vi "2016RefLoopPulseGen_Cleaned.vi"() -> ()   [LabVIEW 2017]
uses:
  <vilib>/Utility/error.llb/DialogType.ctl
  <vilib>/DAQmx/write.llb/DAQmx Write (Digital 1D Bool NChan 1Samp 1Line).vi
  <vilib>/DAQmx/read.llb/DAQmx Read (Analog 1D DBL NChan 1Samp).vi
  <vilib>/DAQmx/write.llb/DAQmx Write (Digital 1D Bool 1Chan 1Samp).vi
  <vilib>/DAQmx/miscellaneous.llb/DAQmx Fill In Error Info.vi
  <vilib>/express/express shared/transition.llb/Dynamic To Waveform Array.vi
  <vilib>/express/express arith-compare/Formula/Block/exnFormulaBlock how many pts in the wave.vi
  <vilib>/express/express shared/ex_Modify Signal Name.vi
  <vilib>/express/express shared/transition.llb/Waveform Array To Dynamic.vi
  <vilib>/DAQmx/create/channels.llb/DAQmx Create Channel (CO-Pulse Generation-Frequency).vi
  <vilib>/DAQmx/configure/timing.llb/DAQmx Timing (Implicit).vi
  <vilib>/DAQmx/configure/timing.llb/DAQmx Timing (Sample Clock).vi
  <vilib>/express/express signal manip/GetorSetDDTAttributes/Set DDT Attributes/SetT0.vi
  <vilib>/express/express arith-compare/Formula/XNode/ExpressFormulaBlockNode.xnode
  <vilib>/express/express signal manip/GetorSetDDTAttributes/Set DDT Attributes/Set DDT Properties.xnode
  <vilib>/addons/control/pid/NI_PID_autopid.lvlib
panel:
  in  "stop 4":bool
  in  "?":bool
  out "error out 2":errorcluster
  out "error out":errorcluster
  in  "output duty cycle range 1":cluster{"output high":dbl, "output low":dbl}={"output high"=100.0, "output low"=0.0}
  out "Waveform Chart":dbl(graph)=1.0280585289001465
  out "Elapsed Time (s)":dbl=1192.0481810569763
  in  "?":T1(tab)
  in  "Lower Test Section offset":dbl
  in  "Vapor Inlet T offset":dbl
  in  "Liquid Tank P offset":dbl=8500.0
  out "Test Section P (Pa)":dbl=116198.57530062649
  in  "P atm":dbl=101325.0
  in  "Liquid Inlet Offset":dbl=1100.0
  in  "Upper Test Sec":dbl
  in  "Dev Section P offset":dbl=-15000.0
  in  "Liquid Inlet T offset":dbl
  in  "Separator T offset":dbl
  in  "Liquid Tank T offset":dbl
  in  "Vapor Tank T offset":dbl
  in  "Separator P Offset":dbl=2500.0
  out "dP [Pa]  W1 to W7":dbl=-0.008208439355650089
  out "dP [Pa] W1 to W4":dbl=0.008075495341450085
  out "Liquid Tank Heater Temp. [C]":dbl=-0.00013997779130803294 format="%#_4g"
  out "Vapor Tank Heater Temp. [C]":dbl=-0.00010921620483495026 format="%#_4g"
  in  "Vapor Tank Heater [V]":dbl(slide) scale=0.0..10.0
  in  "Liquid Tank Heater [V]":dbl(slide) scale=0.0..10.0
  out "Quality\n[-]":dbl=0.5124735258578829 format="%#_3f"
  out "Mixture Enthalpy":dbl=315341.8738601937
  out "Upper TS Sat. Temp. [C]":dbl=-30.741985921320232 format="%#_4g"
  out "Upper Test Section 2\n(not connected)":dbl=19080.10707676887
  out "?":dbl=nan format="%#_4g"
  out "?":dbl=nan format="%#_4g"
  out "Vapor Inlet Sat. Temp. [C]":dbl=18.983650599672455 format="%#_4g"
  out "Liquid Inlet Sat. Temp. [C]":dbl=18.967113726868046 format="%#_4g"
  out "Separator Sat. Temp. [C]":dbl=18.962084458713754 format="%#_4g"
  out "Liquid Tank Sat. Temp. [C]":dbl=17.336038014955804 format="%#_4g"
  out "Vapor Tank Sat. Temp. [C]":dbl=nan format="%#_4g"
  out "Lower Test Section 2\n(not connected)":dbl=-5.945274707393333 format="%#_6f"
  out "Streamwise":dbl=-4309.180034596612 format="%#_2e"
  out "Dev Section":dbl=117529.39865406745 format="%#_5f"
  out "Separator 2":dbl=117436.76445279745 format="%#_5f"
  out "Vapor Tank 2\n(need replaced)":dbl=-34009.73110511369 format="%#_6f"
  out "Liquid Inlet 2":dbl=117458.36040777806 format="%#_5f"
  out "Liquid Tank 2":dbl=119158.55398835387 format="%#_5f"
  out "Upper TS Sat. Pres.":dbl=117745.79282373996
  out "Upper Test Section":dbl=19.02953821278611 format="%#_4g"
  out "Lower Test Section":dbl=18.841711969674257 format="%#_4g"
  out "Vapor Inlet":dbl=19.940090617924646 format="%#_4g"
  out "Liquid Inlet":dbl=19.29273815741822 format="%#_4g"
  out "Separator":dbl=19.351746784304748 format="%#_4g"
  out "Liquid Tank":dbl=19.064732737324512 format="%#_4g"
  out "Vapor Tank":dbl=19.311251471245498 format="%#_4g"
  out "Liquid Inlet Sat. Pres.":dbl=118921.18754866866 format="%#_4f"
  out "Liquid Tank Sat. Pres.":dbl=117902.28866165497 format="%#_4f"
  out "Vapor Inlet Sat. Pres.":dbl=119186.31350697557 format="%#_4f"
  out "Lower Test Section Sat. Pres.":dbl=116914.11104502712 format="%#_4f"
  out "Separator Sat. Pres.":dbl=121862.28710047182 format="%#_4f"
  out "Vapor Tank Sat. Pres.":dbl=119004.3043776936 format="%#_4f"
  out "Evaporator Bottom":dbl=0.07812510710210246 format="%#_4g"
  out "Evaporator Top":dbl=-55440.10937765434 format="%#_4g"
  out "Condenser Bottom":dbl=-0.00013633631982423782 format="%#_4g"
  out "Condenser Top":dbl=-0.0001304783004807413 format="%#_4g"
  in  "Save File":bool
  out "StaticPressDiff(Pa)":dbl=-222.00009683752145
  out "DC":dbl
  out "Vapor Mass Flow Current":dbl=2.098083621149279e-08
  out "Pressure Drop":dbl=2.6226045264365988e-08
  in  "Boolean 2":bool
  out "Waveform Chart 2":dynamicdata(graph)
  in  "Pitot Offset [Pa]":dbl
  in  "PG-TS Offset\n[Pa]":dbl
  in  "Send Pulse 2":bool
  out "Psat liq":dbl=119.96937909943745
  in  "Save Loop Data":bool
  in  "Boolean":bool
  in  "Sampling frequency (Hz)":dbl=1000.0
  in  "Length of recording (s)":dbl=2.0
  in  "PG Abs Offset":dbl=11500.0
  out "Psat vap":dbl=121.24568157832624
  out "Pitot Amps":dbl=2.6415199999999147e-07
  out "dP Pitot Probe":dynamicdata(graph)=[{"t0"=timestamp(3554308544.5452676 s since 1904-01-01), "dt"=0.001, "Y"=array[2000 elements], "attributes"=variant("NI_ChannelName"=variant(string "Pitot dP (Formula Result)"), "NI_OriginalChannelName"=variant(string "Pitot dP"), "NI_UnitDescription"=variant(string "Amps"))}]
  out "Tank Pressure":dynamicdata(graph)=[{"t0"=timestamp(3554308544.5452676 s since 1904-01-01), "dt"=0.001, "Y"=array[2000 elements], "attributes"=variant("NI_ChannelName"=variant(string "Abs P (Formula Result)"), "NI_OriginalChannelName"=variant(string "Abs P"), "NI_UnitDescription"=variant(string "Volts"))}]
  out "dP to test section":dynamicdata(graph)=[{"t0"=timestamp(3554308544.5452814 s since 1904-01-01), "dt"=0.001, "Y"=array[2000 elements], "attributes"=variant("NI_ChannelName"=variant(string "PG to TS dP (Formula Result)"), "NI_OriginalChannelName"=variant(string "PG to TS dP"), "NI_UnitDescription"=variant(string "Volts"))}]
  out "Pitot dP":dbl=-4308.9404273994505
  out "Liquid Temp":dbl=19.52526901660894
  out "Vapor Temp":dbl=19.805676371442082
  in  "CCW":bool
  in  "?":bool
  out "Loop iterations":i32
  in  "Send Pulse":bool
  in  "Steps":i32=10000 min=0 max=40000 step=500
  in  "Idle State":i32(ring)=10214 items=["High"=10192, "Low"=10214]
  in  "Counter(s)":tag="cDAQ1Mod8/ctr0" caption="Counter"
  in  "Duty Cycle":dbl=0.5 min=0.1 max=1.0 step=0.1
  in  "Frequency (Hz)":dbl=1000.0 min=0.0 max=10000.0 step=500.0
  out "Mass Flow Rate":dbl=nan
  in  "Heaters":bool
  out "PG Abs":dbl=119484.80284900061
  out "PG to TS dP":dbl=4351.8068090218785
  in  "Save dP data":bool
  in  "Vapor Flow Set Point [g/s]":dbl format="%.2f"
  in  "stop":bool
  in  "reinitialize? (F) 2":bool=TRUE
  out "Liquid Mass Flow Rate":cluster{"[0]":dbl, "[1]":dbl}(graph)={"[0]"=0.0, "[1]"=-94.2977673785965}
  out "Voltage Out 2":dbl
  out "Liquid Line Density [g/cm3]":dbl=-0.5000013113022632
  out "Liquid Flow Rate [g/s]":dbl=-94.2977673785965
  in  "LiquidOnOff":bool
  in  "LiquidManPID":bool
  in  "PID gains 2":T2={"proportional gain (Kc)"=1e-15, "integral time (Ti, min)"=1e-12, "derivative time (Td, min)"=1e-12} {"derivative time (Td, min)" format="%.4e"; "integral time (Ti, min)" format="%.4e"; "proportional gain (Kc)" format="%.4e"}
  in  "output range 2":cluster{"output high":dbl, "output low":dbl}={"output high"=4.5, "output low"=2.0} {"output low" format="%.2f"; "output high" format="%.2f"}
  in  "Valve Voltage [V] 2":dbl=2.6 format="%.2f"
  in  "Liquid Flow Set Point\n[g/s]":dbl format="%.2f"
  in  "output range":cluster{"output high":dbl, "output low":dbl}={"output high"=3.0, "output low"=2.0} {"output low" format="%.2f"; "output high" format="%.2f"}
  in  "PID gains":T2={"proportional gain (Kc)"=1e-14, "integral time (Ti, min)"=1e-12, "derivative time (Td, min)"=1e-12} {"derivative time (Td, min)" format="%.4e"; "integral time (Ti, min)" format="%.4e"; "proportional gain (Kc)" format="%.4e"}
  in  "VaporManPID":bool
  in  "VaporOnOff":bool
  in  "Valve Voltage [V]":dbl=2.33 format="%.2f"
  out "Vapor Line Density [g/cm3]":dbl=-0.5000029504300922
  out "Vapor Flow Rate [g/s]":dbl=-94.29782933653023
  out "Voltage Out":dbl
  out "Vapor Mass Flow Rate":cluster{"[0]":dbl, "[1]":dbl}(graph)
  in  "reinitialize? (F)":bool=TRUE
  in  "PID on 2":bool
  in  "T1 Setpoint [C]":dbl format="%.2f"
  in  "reinitialize? (F) 3":bool=TRUE
  in  "PID gains 3":T2={"proportional gain (Kc)"=1e-14, "integral time (Ti, min)"=1e-12, "derivative time (Td, min)"=1e-12} {"derivative time (Td, min)" format="%.4e"; "integral time (Ti, min)" format="%.4e"; "proportional gain (Kc)" format="%.4e"}
  out "T1":cluster{"[0]":dbl, "[1]":dbl}(graph)
  out "T1 Measured [C]":dbl
  out "DutyCycleCalc1":dbl format="%.6f"
  in  "T2 Setpoint [C]":dbl format="%.2f"
  in  "reinitialize? (F) 4":bool=TRUE
  in  "PID gains 4":T2={"proportional gain (Kc)"=1e-14, "integral time (Ti, min)"=1e-12, "derivative time (Td, min)"=1e-12} {"derivative time (Td, min)" format="%.4e"; "integral time (Ti, min)" format="%.4e"; "proportional gain (Kc)" format="%.4e"}
  out "T2":cluster{"[0]":dbl, "[1]":dbl}(graph)
  out "T2 Measured [C]":dbl
  out "DutyCycleCalc2":dbl format="%.6f"
  in  "stop 2":bool
  in  "PID on":bool
  in  "PID on 3":bool
  in  "T3 Setpoint [C]":dbl format="%.2f"
  in  "reinitialize? (F) 5":bool=TRUE
  in  "PID gains 5":T2={"proportional gain (Kc)"=1e-14, "integral time (Ti, min)"=1e-12, "derivative time (Td, min)"=1e-12} {"derivative time (Td, min)" format="%.4e"; "integral time (Ti, min)" format="%.4e"; "proportional gain (Kc)" format="%.4e"}
  out "T3":cluster{"[0]":dbl, "[1]":dbl}(graph)
  out "T3 Measured [C]":dbl
  out "DutyCycleCalc3":dbl format="%.6f"
  in  "PID on 4":bool
  in  "T4 Setpoint [C]":dbl format="%.2f"
  in  "reinitialize? (F) 6":bool=TRUE
  in  "PID gains 6":T2={"proportional gain (Kc)"=1e-14, "integral time (Ti, min)"=1e-12, "derivative time (Td, min)"=1e-12} {"derivative time (Td, min)" format="%.4e"; "integral time (Ti, min)" format="%.4e"; "proportional gain (Kc)" format="%.4e"}
  out "T4":cluster{"[0]":dbl, "[1]":dbl}(graph)
  out "T4 Measured [C]":dbl
  out "DutyCycleCalc4":dbl format="%.6f"
  in  "PID on 5":bool
  in  "T5 Setpoint [C]":dbl format="%.2f"
  in  "reinitialize? (F) 7":bool=TRUE
  in  "PID gains 7":T2={"proportional gain (Kc)"=1e-14, "integral time (Ti, min)"=1e-12, "derivative time (Td, min)"=1e-12} {"derivative time (Td, min)" format="%.4e"; "integral time (Ti, min)" format="%.4e"; "proportional gain (Kc)" format="%.4e"}
  out "T5":cluster{"[0]":dbl, "[1]":dbl}(graph)
  out "T5 Measured [C]":dbl
  out "DutyCycleCalc5":dbl format="%.6f"
  in  "PID on 6":bool
  in  "T6 Setpoint [C]":dbl format="%.2f"
  in  "reinitialize? (F) 8":bool=TRUE
  in  "PID gains 8":T2={"proportional gain (Kc)"=1e-14, "integral time (Ti, min)"=1e-12, "derivative time (Td, min)"=1e-12} {"derivative time (Td, min)" format="%.4e"; "integral time (Ti, min)" format="%.4e"; "proportional gain (Kc)" format="%.4e"}
  out "T6":cluster{"[0]":dbl, "[1]":dbl}(graph)
  out "T6 Measured [C]":dbl
  out "DutyCycleCalc6":dbl format="%.6f"
  in  "PID on 7":bool
  in  "T7 Setpoint [C]":dbl format="%.2f"
  in  "reinitialize? (F) 9":bool=TRUE
  in  "PID gains 9":T2={"proportional gain (Kc)"=1e-14, "integral time (Ti, min)"=1e-12, "derivative time (Td, min)"=1e-12} {"derivative time (Td, min)" format="%.4e"; "integral time (Ti, min)" format="%.4e"; "proportional gain (Kc)" format="%.4e"}
  out "T7":cluster{"[0]":dbl, "[1]":dbl}(graph)
  out "T7 Measured [C]":dbl
  out "DutyCycleCalc7":dbl format="%.6f"
  out "WinOn 2":bool
  out "WinOn 1":bool
  in  "PID on 8":bool
  in  "T8 Setpoint [C]":dbl format="%.2f"
  in  "reinitialize? (F) 10":bool=TRUE
  in  "PID gains 10":T2={"proportional gain (Kc)"=1e-14, "integral time (Ti, min)"=1e-12, "derivative time (Td, min)"=1e-12} {"derivative time (Td, min)" format="%.4e"; "integral time (Ti, min)" format="%.4e"; "proportional gain (Kc)" format="%.4e"}
  out "T8":cluster{"[0]":dbl, "[1]":dbl}(graph)
  out "T8 Measured [C]":dbl
  out "DutyCycleCalc8":dbl format="%.6f"
  in  "PID on 9":bool
  in  "T9 Setpoint [C]":dbl format="%.2f"
  in  "reinitialize? (F) 11":bool=TRUE
  in  "PID gains 11":T2={"proportional gain (Kc)"=1e-14, "integral time (Ti, min)"=1e-12, "derivative time (Td, min)"=1e-12} {"derivative time (Td, min)" format="%.4e"; "integral time (Ti, min)" format="%.4e"; "proportional gain (Kc)" format="%.4e"}
  out "T9":cluster{"[0]":dbl, "[1]":dbl}(graph)
  out "T9 Measured [C]":dbl
  out "DutyCycleCalc9":dbl format="%.6f"
  in  "PID on 10":bool
  in  "T10 Setpoint [C]":dbl format="%.2f"
  in  "reinitialize? (F) 12":bool=TRUE
  in  "PID gains 12":T2={"proportional gain (Kc)"=1e-14, "integral time (Ti, min)"=1e-12, "derivative time (Td, min)"=1e-12} {"derivative time (Td, min)" format="%.4e"; "integral time (Ti, min)" format="%.4e"; "proportional gain (Kc)" format="%.4e"}
  out "T10":cluster{"[0]":dbl, "[1]":dbl}(graph)
  out "T10 Measured [C]":dbl
  out "DutyCycleCalc10":dbl format="%.6f"
  in  "PID on 11":bool
  in  "T11 Setpoint [C]":dbl format="%.2f"
  in  "reinitialize? (F) 13":bool=TRUE
  in  "PID gains 13":T2={"proportional gain (Kc)"=1e-14, "integral time (Ti, min)"=1e-12, "derivative time (Td, min)"=1e-12} {"derivative time (Td, min)" format="%.4e"; "integral time (Ti, min)" format="%.4e"; "proportional gain (Kc)" format="%.4e"}
  out "T11":cluster{"[0]":dbl, "[1]":dbl}(graph)
  out "T11 Measured [C]":dbl
  out "DutyCycleCalc11":dbl format="%.6f"
  in  "PID on 12":bool
  in  "T12 Setpoint [C]":dbl format="%.2f"
  in  "reinitialize? (F) 14":bool=TRUE
  in  "PID gains 14":T2={"proportional gain (Kc)"=1e-14, "integral time (Ti, min)"=1e-12, "derivative time (Td, min)"=1e-12} {"derivative time (Td, min)" format="%.4e"; "integral time (Ti, min)" format="%.4e"; "proportional gain (Kc)" format="%.4e"}
  out "T12":cluster{"[0]":dbl, "[1]":dbl}(graph)
  out "T12 Measured [C]":dbl
  out "DutyCycleCalc12":dbl format="%.6f"
  in  "PID on 13":bool
  in  "T13 Setpoint [C]":dbl format="%.2f"
  in  "reinitialize? (F) 15":bool=TRUE
  in  "PID gains 15":T2={"proportional gain (Kc)"=1e-14, "integral time (Ti, min)"=1e-12, "derivative time (Td, min)"=1e-12} {"derivative time (Td, min)" format="%.4e"; "integral time (Ti, min)" format="%.4e"; "proportional gain (Kc)" format="%.4e"}
  out "T13":cluster{"[0]":dbl, "[1]":dbl}(graph)
  out "T13 Measured [C]":dbl
  out "DutyCycleCalc13":dbl format="%.6f"
  in  "PID on 14":bool
  in  "T14 Setpoint [C]":dbl format="%.2f"
  in  "reinitialize? (F) 16":bool=TRUE
  in  "PID gains 16":T2={"proportional gain (Kc)"=1e-14, "integral time (Ti, min)"=1e-12, "derivative time (Td, min)"=1e-12} {"derivative time (Td, min)" format="%.4e"; "integral time (Ti, min)" format="%.4e"; "proportional gain (Kc)" format="%.4e"}
  out "T14":cluster{"[0]":dbl, "[1]":dbl}(graph)
  out "T14 Measured [C]":dbl
  out "DutyCycleCalc14":dbl format="%.6f"
  # "Same button as Save data loop button on Pulse Generator tab"
  # "Test Section Properties"
  # "Pressure\n[Pa]"
  # "Sat. Temp.\n[C]"
  # "Sat. Pressure\n[Pa]"
  # "Temp.\n[C]"
  # "Temperature [C]"
  # "Condenser"
  # "Evaporator"
  # "Top"
  # "Bottom"
  # "Save File"
  # "Do Not\nSave File"
  # "In order to send a  group of pulses follow the steps below.\n1)Press the button labeled Send Pulse\n2)Press the button a second time in order to prepare for another pulse\n3)Press the stop button to reset the Send Pulse button\n4)Repeat process for next pulse\n\nNote: 1000 steps is a full cycle of the valve, this will send one pulse"
  # "Saving Data:\n\n- Press the Save Loop Data button to record time-averaged (every 2s) data from the loop (data from Test Section Properties tab). Pressing the button again keeps writing in the same file.\n\n-Press the Save dP data to record time resolved data. Each time you press the button, a new file is recorded."
  # "Pulse Generator\nTemperatures"
  # "Vapor Side"
  # "Valve On"
  # "Valve Off"
  # "Manual Flow\nControl"
  # "PID Flow\nControl"
  # "Liquid Side"
  # "Valve On"
  # "Valve Off"
  # "Manual Flow\nControl"
  # "PID Flow\nControl"
  # "Heater On"
  # "Heater On"
  # "Heater On"
  # "Heater On"
  # "Heater Off"
  # "Heater Off"
  # "Heater Off"
  # "Heater Off"
  # "Heater On"
  # "Heater On"
  # "Heater On"
  # "Heater Off"
  # "Heater Off"
  # "Heater Off"
  # "Heater On"
  # "Heater On"
  # "Heater On"
  # "Heater On"
  # "Heater Off"
  # "Heater Off"
  # "Heater Off"
  # "Heater Off"
  # "Heater On"
  # "Heater On"
  # "Heater On"
  # "Heater Off"
  # "Heater Off"
  # "Heater Off"
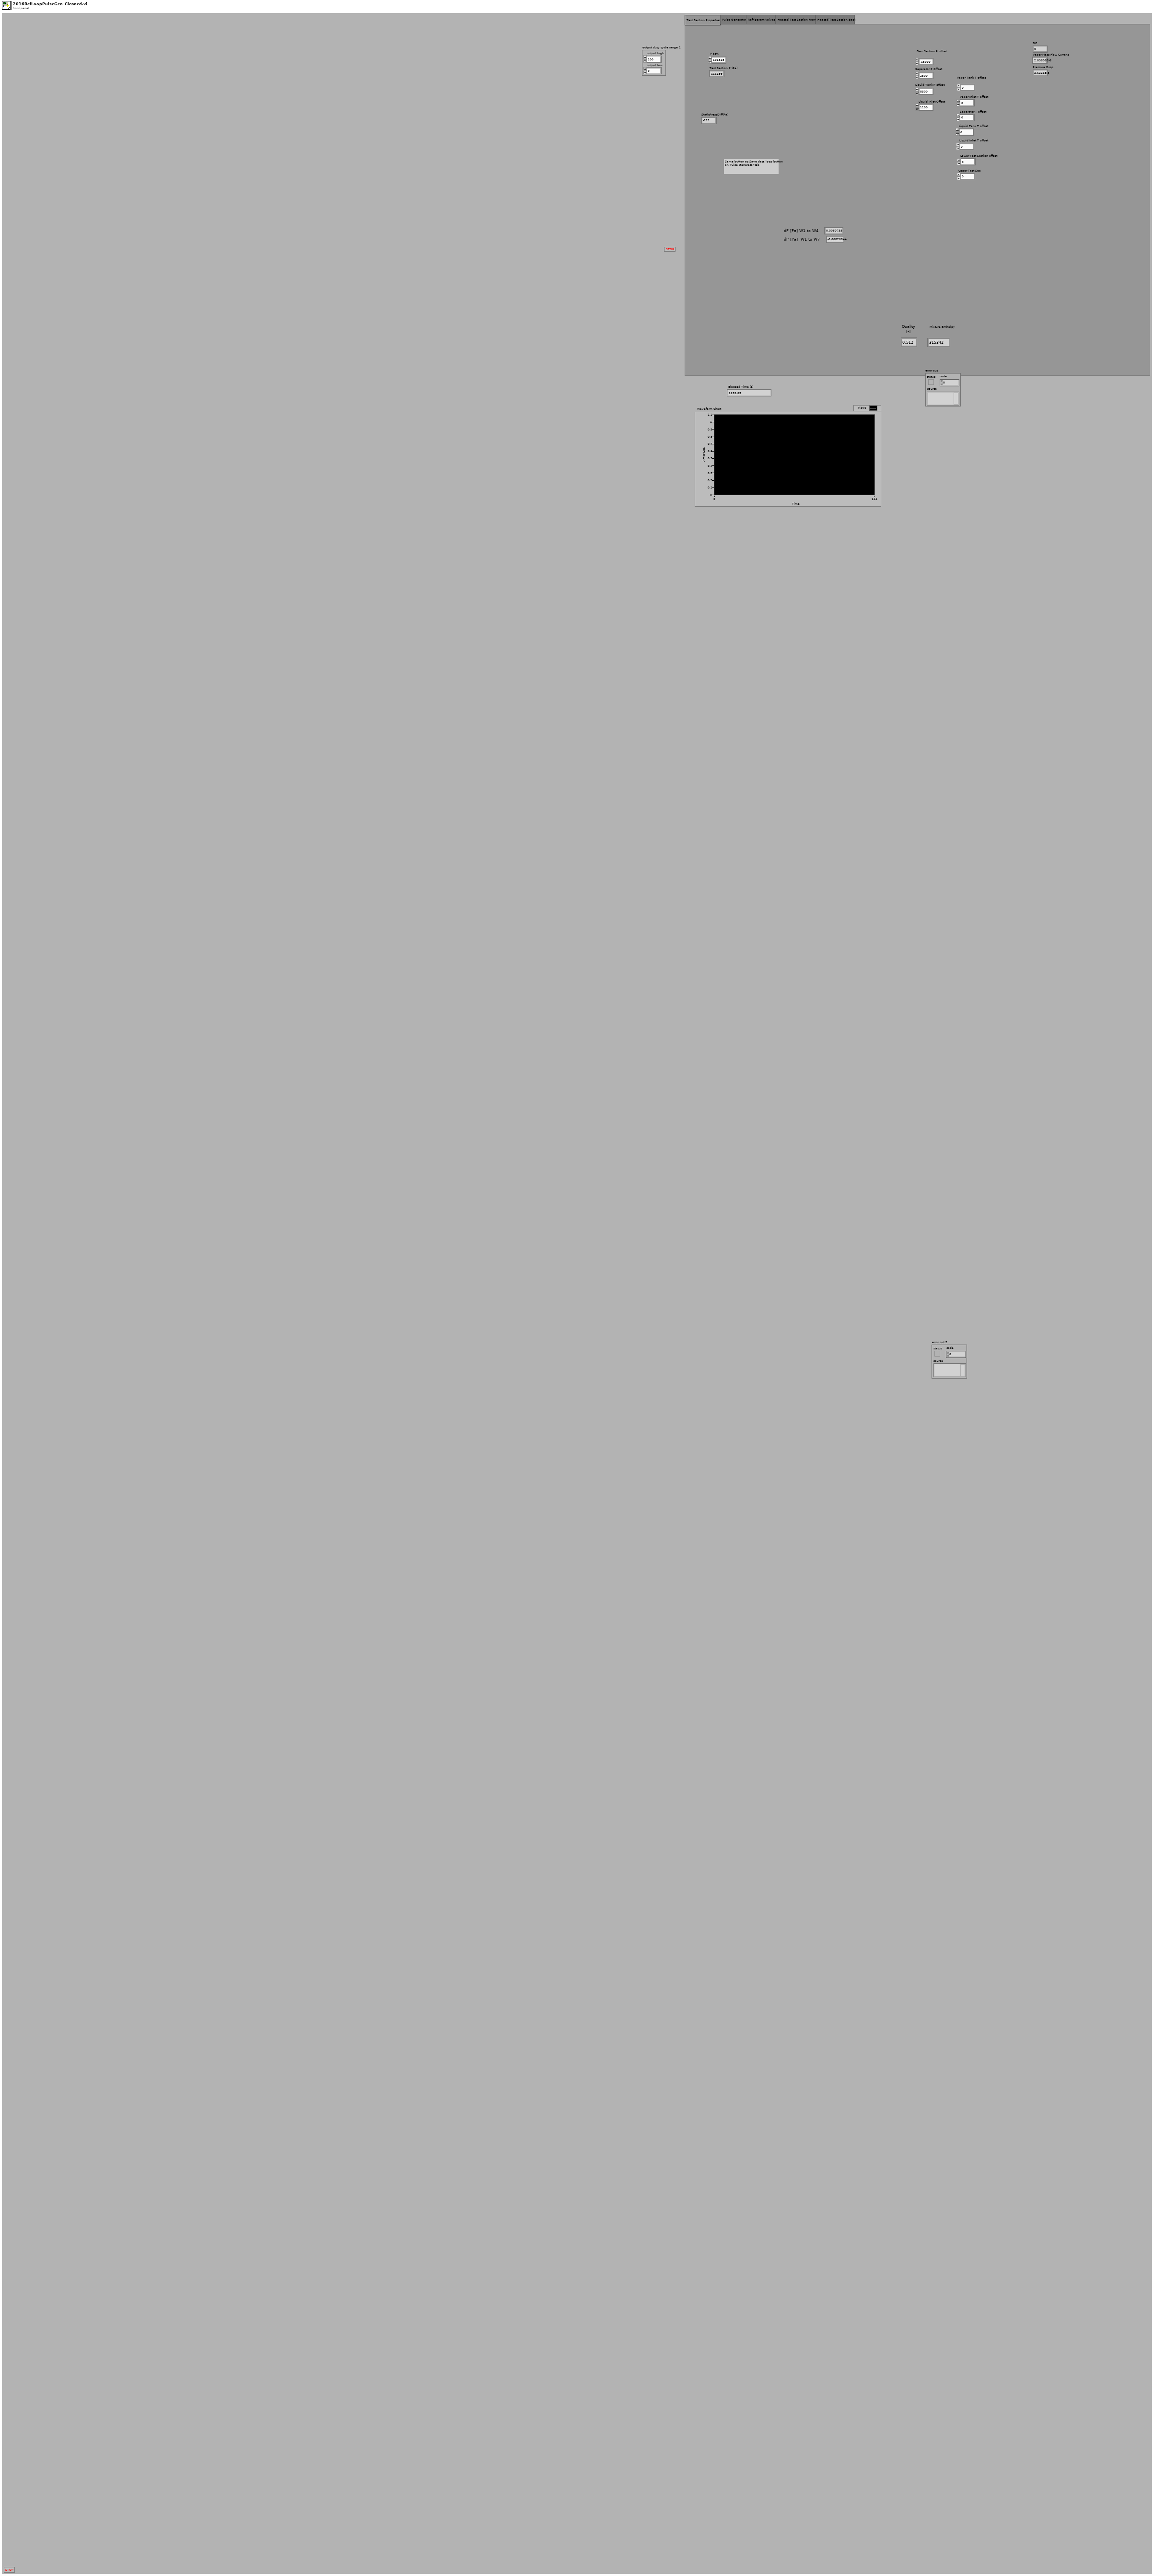
[diagram p1: front panel]
types:
  T1 = enum32{"Test Section Properties", "Pulse Generator", "Refrigerant Valves", "Heated Test Section Front", "Heated Test Section Back"}
  T2 = cluster{"proportional gain (Kc)":dbl, "integral time (Ti, min)":dbl, "derivative time (Td, min)":dbl}
  T3 = typedef "DialogType.ctl" = u16
  T4 = cluster{bool[], bool[], bool[], bool[], bool[], bool[], bool[], bool[], bool[], bool[], bool[], bool[], bool[], bool[]}
  T5 = cluster{"controller type":u16, "relay cycles":i32, "relay amplitude":dbl, "control specification":u16, "PV noise level":dbl}
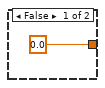
[diagram p6: hidden frame]
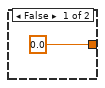
[diagram p7: hidden frame]
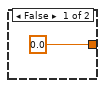
[diagram p8: hidden frame]
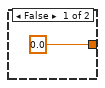
[diagram p9: hidden frame]
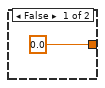
[diagram p10: hidden frame]
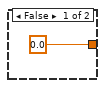
[diagram p11: hidden frame]
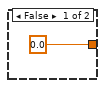
[diagram p12: hidden frame]
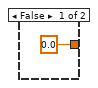
[diagram p13: hidden frame]
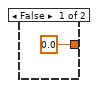
[diagram p14: hidden frame]
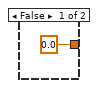
[diagram p15: hidden frame]
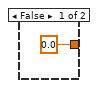
[diagram p16: hidden frame]
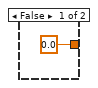
[diagram p17: hidden frame]
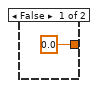
[diagram p18: hidden frame]
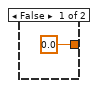
[diagram p19: hidden frame]
diagram:
  w1 = T3 3 items=["no dialog", "OK message", "continue or stop message", "OK message + warnings", "continue/stop + warnings"] ("type of dialog (OK msg:1)")
  w11 = refnum<k21> "DigitalTaskOut1"  # DAQmx Task Name
  w19 = refnum<k21> "HeatedTSWindows"  # DAQmx Task Name
  n1 = while {
    stop <- "stop" stop-if-true
    # "Window 3-4 P"
    # "Need to add new pressure sensor on test seciton"
    # "Dev Section P"
    # "liq inlet"
    # "sep tk"
    # "liq tk"
    # "vapor tk"
    # "Calibrations used by Mark for thermocouples:\nIn temp vapor tank:\n(24642*V)+24.36\nIn temp liquid tank:\n(24869*V)+24.24\nIn temp liquid inlet:\n(24775*V)+24.24\nIn temp vapor inlet:\n(24515*V)+24.29"
    n2 = call "DAQ Assistant3"() -> ("data"=w198:dynamicdata)  [unwired: 17 in, 2 out]
    n3 = Split Signals(w198) -> (w74:dynamicdata, w124:dynamicdata, w73:dynamicdata, w97:dynamicdata, w45:dynamicdata, w39:dynamicdata, w197:dynamicdata, w196:dynamicdata, w139:dynamicdata, w199:dynamicdata, w200:dynamicdata, w201:dynamicdata, w202:dynamicdata, w203:dynamicdata, w195:dynamicdata, w194:dynamicdata, w189:dynamicdata, w188:dynamicdata, w186:dynamicdata, w138:dynamicdata, w137:dynamicdata, w128:dynamicdata, w127:dynamicdata, w126:dynamicdata, w125:dynamicdata, w72:dynamicdata)  [unwired: 26 in]
    "Vapor Mass Flow Current" <- w74
    "Pressure Drop" <- w186
    n4 = call "GagePressure.vi"("Abs. Pressure\nVoltage [V]"=w72) -> ("Absolute Pressure [kPa]"=w71:dbl)  [unwired: 10 in]
    n5 = call "UpperTSPres.vi"("Abs. Pressure\nVoltage [V]"=w137) -> ("Absolute Pressure [kPa]"=w122:dbl)  [unwired: 10 in]
    "Upper Test Section 2\n(not connected)" <- w122
    n6 = call "TemperatureVaporTank.vi"("Temp. Voltage\n[V]"=w128) -> ("Temp. []"=w131:dbl)  [unwired: 10 in]
    "Condenser Top" <- w131
    n7 = call "TemperatureVaporTank.vi"("Temp. Voltage\n[V]"=w127) -> ("Temp. []"=w130:dbl)  [unwired: 10 in]
    "Condenser Bottom" <- w130
    n8 = call "TemperatureVaporTank.vi"("Temp. Voltage\n[V]"=w126) -> ("Temp. []"=w129:dbl)  [unwired: 10 in]
    "Evaporator Top" <- w129
    n9 = call "TemperatureVaporTank.vi"("Temp. Voltage\n[V]"=w125) -> ("Temp. []"=w79:dbl)  [unwired: 10 in]
    "Evaporator Bottom" <- w79
    n10 = call "AbsolutePressure.vi"("Abs. Pressure\nVoltage [V]"=w195) -> ("Absolute Pressure [kPa]"=w184:dbl)  [unwired: 10 in]
    "Lower Test Section 2\n(not connected)" <- w184
    n11 = call "TemperatureVaporTank.vi"("Temp. Voltage\n[V]"=w138) -> ("Temp. []"=w82:dbl)  [unwired: 10 in]
    n12 = call "VapTankVapInPressure.vi"("Abs. Pressure\nVoltage [V]"=w39) -> ("Absolute Pressure [kPa]"=w38:dbl)
    n13 = call "SepLiqInPressure.vi"("Abs. Pressure\nVoltage [V]"=w197) -> ("Absolute Pressure [kPa]"=w36:dbl)
    n14 = call "TemperatureVaporInlet.vi"("Temp. Voltage\n[V]"=w200) -> ("Temp. []"=w66:dbl)  [unwired: 10 in]
    n15 = call "TemperatureVaporTank.vi"("Temp. Voltage\n[V]"=w203) -> ("Temp. []"=w89:dbl)  [unwired: 10 in]
    n16 = call "TemperatureVaporTank.vi"("Temp. Voltage\n[V]"=w194) -> ("Temp. []"=w34:dbl)  [unwired: 10 in]
    n17 = Add(x="P atm", y=w71) -> (x+y=w69:dbl)
    "Test Section P (Pa)" <- w69
    n18 = xnode ("Output Current to Flow")("I"=w74) -> ("Result"=w113:dynamicdata)  [unwired: 1 in, 1 out]
    n19 = xnode ("Vapor Line Density")("DensCurr"=w124) -> ("Result"=w107:dynamicdata)  [unwired: 1 in, 1 out]
    n20 = xnode ("Output Current to Flow 2")("I"=w73) -> ("Result"=w105:dynamicdata)  [unwired: 1 in, 1 out]
    n21 = xnode ("Liquid Line Density")("DensCurr"=w97) -> ("Result"=w102:dynamicdata)  [unwired: 1 in, 1 out]
    n22 = Add(x=w89, y="Separator T offset") -> (x+y=w84:dbl)
    "Vapor Inlet" <- w84
    n23 = call "TemperatureLiquidInlet.vi"("Temp. Voltage\n[V]"=w202) -> ("Temp. [C]"=w42:dbl)  [unwired: 10 in]
    n24 = xnode "Formula"("P"=w38) -> ("Result"=w159:dbl)  [unwired: 1 in, 1 out]
    n25 = Add(x=w82, y="Upper Test Sec") -> (x+y=w80:dbl)
    "Upper Test Section" <- w80
    n26 = call "PressureChange.vi"("Pressure Voltage (V)"=w186) -> ("Streamwise dP (kPa)"=w76:dbl)  [unwired: 10 in]
    "Streamwise" <- w76
    n27 = Add(x=w66, y="Vapor Inlet T offset") -> (x+y=w64:dbl)
    "Separator" <- w64
    n28 = To Double Precision Float(number=w107) -> (double precision float=→"Vapor Line Density [g/cm3]":dbl)
    n29 = call "Statistics"("Signals"=w113) -> ("Arithmetic Mean"=w98:dynamicdata)  [unwired: 25 in, 1 out]
    n30 = call "Statistics2"("Signals"=w105) -> ("Arithmetic Mean"=w47:dynamicdata)  [unwired: 25 in, 1 out]
    n31 = To Double Precision Float(number=w102) -> (double precision float=→"Liquid Line Density [g/cm3]":dbl)
    n32 = Add(x=w80, y=273.15) -> (x+y=w132:dbl)
    n33 = Subtract(x=w159, y=0.0) -> (x-y=→"Liquid Tank Sat. Temp. [C]":dbl)
    n34 = Add(x=259.15, y=w42) -> (x+y=w178:dbl)
    n35 = call "TemperatureLiquidTank.vi"("Temp. Voltage\n[V]"=w201) -> ("Temp. []"=w91:dbl)  [unwired: 10 in]
    n36 = Add(x=w34, y="Lower Test Section offset") -> (x+y=w30:dbl)
    "Lower Test Section" <- w30
    n37 = call "TemperatureVaporTank.vi"("Temp. Voltage\n[V]"=w189) -> ("Temp. []"=w185:dbl)  [unwired: 10 in]
    "Vapor Tank Heater Temp. [C]" <- w185
    n38 = call "TemperatureVaporTank.vi"("Temp. Voltage\n[V]"=w188) -> ("Temp. []"=w187:dbl)  [unwired: 10 in]
    "Liquid Tank Heater Temp. [C]" <- w187
    n39 = Add(x=w36, y="Separator P Offset") -> (x+y=w78:dbl)
    "Separator 2" <- w78
    n40 = call "VapTankVapInPressure.vi"("Abs. Pressure\nVoltage [V]"=w45) -> ("Absolute Pressure [kPa]"=w43:dbl)
    "Vapor Tank 2\n(need replaced)" <- w43
    n41 = call "Convert from Dynamic Data2"("Dynamic Data Type"=w47, "Channel"=0) -> ("Scalar"=w58:dbl)  [unwired: 2 in]
    "Liquid Flow Rate [g/s]" <- w58
    n42 = Add(x=w38, y="Liquid Tank P offset") -> (x+y=w67:dbl)
    "Liquid Tank 2" <- w67
    n43 = call "Convert from Dynamic Data"("Dynamic Data Type"=w98, "Channel"=0) -> ("Scalar"=w28:dbl)  [unwired: 2 in]
    "Vapor Flow Rate [g/s]" <- w28
    n44 = call "SepLiqInPressure.vi"("Abs. Pressure\nVoltage [V]"=w196) -> ("Absolute Pressure [kPa]"=w51:dbl)
    n45 = call "VapIn.vi"("Abs. Pressure\nVoltage [V]"=w139) -> ("Absolute Pressure [kPa]"=w77:dbl)  [unwired: 10 in]
    n46 = call "TemperatureVaporTank.vi"("Temp. Voltage\n[V]"=w199) -> ("Temp. []"=w75:dbl)  [unwired: 10 in]
    n47 = Add(x=273.15, y=w30) -> (x+y=w167:dbl)
    n48 = xnode "Formula"("P"=w184) -> ("Result"=w149:dbl)  [unwired: 1 in, 1 out]
    n49 = xnode "Formula"("T"=w167) -> ("Result"=w116:dbl)  [unwired: 1 in, 1 out]
    "Lower Test Section Sat. Pres." <- w116
    n50 = xnode "Formula"("T"=w132) -> ("Result"=w115:dbl)  [unwired: 1 in, 1 out]
    "Upper TS Sat. Pres." <- w115
    n51 = xnode "Formula"("P"=w122) -> ("Result"=w136:dbl)  [unwired: 1 in, 1 out]
    n52 = xnode "Formula"("P"=w76) -> ("Result"=w146:dbl)  [unwired: 1 in, 1 out]
    n53 = xnode "Formula"("T_v"=w64, "P_v"=w77) -> ("Result"=w141:dbl)  [unwired: 1 in, 1 out]
    n54 = xnode "Formula"("T"=w178) -> ("Result"=w143:dbl)  [unwired: 1 in, 1 out]
    n55 = Add(x=273.15, y=w64) -> (x+y=w169:dbl)
    n56 = Subtract(x=w149, y=0.0) -> (x-y=→"?":dbl)
    n57 = Add(x=w42, y="Liquid Inlet T offset") -> (x+y=w40:dbl)
    "Liquid Inlet" <- w40
    n58 = Subtract(x=w136, y=0.0) -> (x-y=→"Upper TS Sat. Temp. [C]":dbl)
    n59 = Build Array(w28, "Vapor Flow Set Point [g/s]") -> (w61:dbl[])
    n60 = Subtract(x=w146, y=0.0) -> (x-y=→"?":dbl)
    n61 = Merge Signals(w28, w58, w43, w67, w78, w51, w77, w76, w75, w64, w91, w42, w84, w184, w30, w185, w187, w82, w122, w131, w130, w129, w79, w69) -> (w123:dynamicdata)
    n62 = Add(x=273.15, y=w84) -> (x+y=w165:dbl)
    n63 = Array To Cluster(array=w61) -> (cluster=→"Vapor Mass Flow Rate":cluster{"[0]":dbl, "[1]":dbl})
    n64 = case shown="True" "Save File" {
      tunnel: w123 -> [_ w518]
      frame False {
      }
      frame True {
        n65 = call "Write To Measurement File"("Signals"=w518) -> ()  [unwired: 16 in, 3 out]
      }
    }
    n66 = case shown="False" "VaporManPID" {
      tunnel: [w511 w517] -> w110
      tunnel: w28 -> [w509 _]
      tunnel: "Valve Voltage [V]" -> [w505 w517]
      tunnel: "Vapor Flow Set Point [g/s]" -> [w508 _]
      frame False {
        n67 = call <vilib>:"PID Autotuning.vi"("reinitialize? (F)"="reinitialize? (F)", "PID gains"="PID gains", "process variable"=w508, "setpoint"=w509) -> ("output"=w507:dbl)  [unwired: 4 in, 3 out]
        n68 = Cluster To Array(cluster="output range") -> (array=w514:dbl[])
        n69 = Add(x=w507, y=w505) -> (x+y=w506:dbl)
        n70 = Array Max & Min(array=w514) -> (max value=w513:dbl, min value=w512:dbl)  [unwired: 2 out]
        n71 = In Range and Coerce(upper limit=w513, x=w506, lower limit=w512) -> (coerced(x)=w511:dbl)  [unwired: 1 out]
      }
      frame True {
      }
    }
    n72 = Subtract(x=w116, y=w115) -> (x-y=w121:dbl)
    n73 = Divide(x=w121, y=2.54) -> (x/y=w119:dbl)
    n74 = Multiply(x=w119, y=0.678) -> (x*y=→"StaticPressDiff(Pa)":dbl)
    n75 = xnode "Formula"("P"=w43) -> ("Result"=w44:dbl)  [unwired: 1 in, 1 out]
    n76 = xnode "Formula"("P"=w78) -> ("Result"=w52:dbl)  [unwired: 1 in, 1 out]
    n77 = Build Array(w58, "Liquid Flow Set Point\n[g/s]") -> (w99:dbl[])
    n78 = case shown="False" "LiquidManPID" {
      tunnel: "Liquid Flow Set Point\n[g/s]" -> [w363 _]
      tunnel: [w355 w365] -> w54
      tunnel: w58 -> [w362 _]
      tunnel: "Valve Voltage [V] 2" -> [w354 w365]
      frame False {
        n79 = call <vilib>:"PID Autotuning.vi"("reinitialize? (F)"="reinitialize? (F) 2", "PID gains"="PID gains 2", "process variable"=w362, "setpoint"=w363) -> ("output"=w361:dbl)  [unwired: 4 in, 3 out]
        n80 = Cluster To Array(cluster="output range 2") -> (array=w358:dbl[])
        n81 = Add(x=w354, y=w361) -> (x+y=w360:dbl)
        n82 = Array Max & Min(array=w358) -> (max value=w356:dbl, min value=w357:dbl)  [unwired: 2 out]
        n83 = In Range and Coerce(upper limit=w356, x=w360, lower limit=w357) -> (coerced(x)=w355:dbl)  [unwired: 1 out]
      }
      frame True {
      }
    }
    n84 = xnode "Formula"("m_dot_l"=w58, "h_l"=w143, "m_dot_v"=w28, "h_v"=w141) -> ("Result"=w144:dbl)  [unwired: 1 in, 1 out]
    "Mixture Enthalpy" <- w144
    n85 = xnode "Formula"("T"=w169) -> ("Result"=→"Vapor Inlet Sat. Pres.":dbl)  [unwired: 1 in, 1 out]
    n86 = xnode "Formula"("T"=w165) -> ("Result"=→"Separator Sat. Pres.":dbl)  [unwired: 1 in, 1 out]
    n87 = Add(x=w51, y="Liquid Inlet Offset") -> (x+y=w49:dbl)
    "Liquid Inlet 2" <- w49
    n88 = Add(x=w75, y="Vapor Tank T offset") -> (x+y=w85:dbl)
    "Vapor Tank" <- w85
    n89 = Add(x=w77, y="Dev Section P offset") -> (x+y=w63:dbl)
    "Dev Section" <- w63
    n90 = Add(x="Liquid Tank T offset", y=w91) -> (x+y=w86:dbl)
    "Liquid Tank" <- w86
    n91 = Array To Cluster(array=w99) -> (cluster=→"Liquid Mass Flow Rate":cluster{"[0]":dbl, "[1]":dbl})
    n92 = Subtract(x=w44, y=0.0) -> (x-y=→"Vapor Tank Sat. Temp. [C]":dbl)
    n93 = Subtract(x=w52, y=0.0) -> (x-y=→"Separator Sat. Temp. [C]":dbl)
    n94 = Add(x=273.15, y=w64) -> (x+y=w175:dbl)
    n95 = xnode "Formula"("T"=w175) -> ("Result"=w142:dbl)  [unwired: 1 in, 1 out]
    n96 = Add(x=273.15, y=w40) -> (x+y=w173:dbl)
    n97 = xnode "Formula"("P"=w49) -> ("Result"=w154:dbl)  [unwired: 1 in, 1 out]
    n98 = case shown="False" "Boolean 2" {
      tunnel: w28 -> [w209 w212]
      tunnel: w58 -> [w210 w213]
      tunnel: [w210 w213] -> w32
      tunnel: [w209 w212] -> w33
      tunnel: w63 -> [w208 w211]
      tunnel: [w208 w211] -> w31
      frame False {
      }
      frame True {
      }
    }
    n99 = xnode "Formula"("P"=w63) -> ("Result"=w83:dbl)  [unwired: 1 in, 1 out]
    n100 = xnode "Formula"("h_mix"=w144, "h_l"=w143, "h_v"=w142) -> ("Result"=→"Quality\n[-]":dbl)  [unwired: 1 in, 1 out]
    n101 = xnode "Formula"("T"=w173) -> ("Result"=→"Liquid Inlet Sat. Pres.":dbl)  [unwired: 1 in, 1 out]
    n102 = Add(x=273.15, y=w85) -> (x+y=w163:dbl)
    n103 = Add(x=273.15, y=w86) -> (x+y=w171:dbl)
    n104 = xnode "Formula"("T"=w163) -> ("Result"=→"Vapor Tank Sat. Pres.":dbl)  [unwired: 1 in, 1 out]
    n105 = xnode "Formula"("T"=w171) -> ("Result"=→"Liquid Tank Sat. Pres.":dbl)  [unwired: 1 in, 1 out]
    n106 = Subtract(x=w154, y=0.0) -> (x-y=→"Liquid Inlet Sat. Temp. [C]":dbl)
    n107 = Subtract(x=w83, y=0.0) -> (x-y=→"Vapor Inlet Sat. Temp. [C]":dbl)
    n108 = Merge Signals(w33, w32, w31) -> (w27:dynamicdata)
    n109 = call "Write To Measurement File3"("Signals"=w27, "Enable"=FALSE) -> ()  [unwired: 15 in, 3 out]
    n110 = Boolean To (0,1)(Boolean="VaporOnOff") -> (0, 1=w111:i16)
    n111 = Boolean To (0,1)(Boolean="LiquidOnOff") -> (0, 1=w103:i16)
    n112 = To Double Precision Float(number=w111) -> (double precision float=w109:dbl)
    n113 = To Double Precision Float(number=w103) -> (double precision float=w59:dbl)
    n114 = Multiply(x=w54, y=w59) -> (x*y=w53:dbl)
    "Voltage Out 2" <- w53
    n115 = xnode "Formula"("V"="Liquid Tank Heater [V]") -> ("Result"=w205:dbl)  [unwired: 1 in, 1 out]
    n116 = xnode "Formula"("V"="Vapor Tank Heater [V]") -> ("Result"=w204:dbl)  [unwired: 1 in, 1 out]
    n117 = Multiply(x=w110, y=w109) -> (x*y=w108:dbl)
    "Voltage Out" <- w108
    n118 = call "Simulate Signal4"("Offset"=w53) -> ("DC"=w192:dynamicdata)  [unwired: 13 in, 1 out]
    n119 = call "Simulate Signal3"("Offset"=w108) -> ("DC"=w193:dynamicdata)  [unwired: 13 in, 1 out]
    n120 = call "Simulate Signal"("Offset"=w205) -> ("DC"=w191:dynamicdata)  [unwired: 13 in, 1 out]
    n121 = call "Simulate Signal2"("Offset"=w204) -> ("DC"=w190:dynamicdata)  [unwired: 13 in, 1 out]
    "DC" <- w190
    n122 = Merge Signals(w192, w193, w190, w191) -> (w94:dynamicdata)
    n123 = call "DAQ Assistant"("data"=w94) -> ()  [unwired: 17 in, 2 out]
  }
  n124 = while {
    tunnel: [w1004] -> w2
    stop <- "?" stop-if-true
    w996 = 10178 items=["Continuous Samples"=10123, "Finite Samples"=10178]
    n125 = Merge Signals("CCW", "Heaters") -> (w988:dynamicdata)
    n126 = call "Convert from Dynamic Data3"("Dynamic Data Type"=w988) -> ("Array"=w987:bool[])  [unwired: 3 in]
    n127 = call-poly <vilib>:"DAQmx Create Virtual Channel.vi"("frequency"="Frequency (Hz)", "duty cycle"="Duty Cycle", "counter"="Counter(s)", "idle state"="Idle State", "initial delay"=0.0) -> ("task out"=w998:refnum<k21>, "error out"=w997:errorcluster)  [unwired: 9 in]
    n128 = call "DAQ Assistant4"("data"=w987) -> ()  [unwired: 17 in, 2 out]
    n129 = call-poly <vilib>:"DAQmx Timing.vi"("task/channels in"=w998, "sample mode"=w996, "samples per channel"="Steps", "error in"=w997) -> ("task out"=w992:refnum<k21>, "error out"=w991:errorcluster)  [unwired: 10 in]
    n130 = case shown="True" "Send Pulse" {
      tunnel: [w1005 w1012] -> w994
      tunnel: [w1006 w1011] -> w993
      tunnel: w992 -> [w1006 w1008]
      tunnel: w991 -> [w1005 w1007]
      frame False {
      }
      frame True {
        n131 = call <vilib>:"DAQmx Start Task.vi"("task/channels in"=w1008, "error in"=w1007) -> ("task out"=w1010:refnum<k21>, "error out"=w1009:errorcluster)  [unwired: 12 in]
        n132 = while {
          tunnel: w1010 -> [w1020]
          tunnel: w1009 -> [w1019]
          tunnel: [w1016] -> w1011
          tunnel: [w1015] -> w1012
          i -> [w1014]
          stop <- w1017 stop-if-true
          n133 = call <vilib>:"DAQmx Is Task Done.vi"("task/channels in"=w1020, "error in"=w1019) -> ("task out"=w1016:refnum<k21>, "error out"=w1015:errorcluster)  [unwired: 11 in, 1 out]
          n134 = Unbundle By Name(w1015) -> ("status"=w1018:bool)
          n135 = Or(x=w1018, y="?") -> (x .or. y?=w1017:bool)
          "Loop iterations" <- w1014
        }
      }
    }
    n136 = call <vilib>:"DAQmx Clear Task.vi"("task in"=w993, "error in"=w994) -> ("error out"=w1004:errorcluster)  [unwired: 13 in]
  }
  n137 = while {
    stop <- "stop 4" stop-if-true
    n138 = local write "Send Pulse"("Send Pulse 2") -> ()
    n139 = local write "Save File"("Save Loop Data") -> ()
    n140 = Multiply(x="Length of recording (s)", y="Sampling frequency (Hz)") -> (x*y=w1038:dbl)
    n141 = call "DAQ Assistant6"("rate"="Sampling frequency (Hz)", "number of samples"=w1038) -> ("task out"=w1040:refnum<k21>, "data"=w1061:dynamicdata)  [unwired: 14 in, 2 out]
    n142 = Split Signals(w1061) -> (w1049:dynamicdata, w1063:dynamicdata, w1060:dynamicdata, w1046:dynamicdata, w1031:dynamicdata, w1033:dynamicdata, w1032:dynamicdata, →"Waveform Chart 2":dynamicdata)  [unwired: 8 in]
    "Vapor Temp" <- w1046
    "Liquid Temp" <- w1031
    "Pitot Amps" <- w1060
    n143 = case shown="True" "Boolean" {
      tunnel: w1040 -> [_ w1485]
      tunnel: "Sampling frequency (Hz)" -> [_ w1483]
      tunnel: w1038 -> [_ w1482]
      frame False {
      }
      frame True {
        n144 = call <vilib>:"DAQmx Stop Task.vi"("task/channels in"=w1485) -> ("task out"=w1484:refnum<k21>)  [unwired: 13 in, 1 out]
        n145 = call-poly <vilib>:"DAQmx Timing.vi"("task/channels in"=w1484, "samples per channel"=w1482, "rate"=w1483) -> ()  [unwired: 11 in, 2 out]
      }
    }
    n146 = xnode "Formula"("V"=w1049) -> ("Result"=w1055:dynamicdata)  [unwired: 1 in, 1 out]
    n147 = xnode "Formula"("V"=w1063) -> ("Result"=w1027:dynamicdata)  [unwired: 1 in, 1 out]
    n148 = xnode "Formula"("T"=w1046) -> ("Result"=→"Psat vap":dynamicdata)  [unwired: 1 in, 1 out]
    n149 = xnode "Formula"("I"=w1060) -> ("Result"=w1022:dynamicdata)  [unwired: 1 in, 1 out]
    n150 = xnode "Formula"("T"=w1031) -> ("Result"=→"Psat liq":dynamicdata)  [unwired: 1 in, 1 out]
    n151 = xnode "Formula"("I"=w1033) -> ("Result"=→"dP [Pa] W1 to W4":dynamicdata)  [unwired: 1 in, 1 out]
    n152 = xnode "Formula"("I"=w1032) -> ("Result"=→"dP [Pa]  W1 to W7":dynamicdata)  [unwired: 1 in, 1 out]
    n153 = xnode "Formula"("T"=w1046) -> ("Result"=w1064:dynamicdata)  [unwired: 1 in, 1 out]
    n154 = xnode "Formula"("P"=w1022) -> ("Result"=w1062:dynamicdata)  [unwired: 1 in, 1 out]
    n155 = xnode "Formula"("P"=w1022) -> ("Result"=w1024:dynamicdata)  [unwired: 1 in, 1 out]
    n156 = xnode "Formula"("dP"=w1062, "rho"=w1064) -> ("Result"=w1058:dynamicdata)  [unwired: 1 in, 1 out]
    "Mass Flow Rate" <- w1058
    n157 = Add(x="PG-TS Offset\n[Pa]", y=w1027) -> (x+y=w1026:dynamicdata)
    "PG to TS dP" <- w1026
    "dP to test section" <- w1026
    n158 = Add(x="PG Abs Offset", y=w1055) -> (x+y=w1052:dynamicdata)
    "PG Abs" <- w1052
    "Tank Pressure" <- w1052
    n159 = Add(x="Pitot Offset [Pa]", y=w1024) -> (x+y=w1023:dynamicdata)
    "Pitot dP" <- w1023
    "dP Pitot Probe" <- w1023
    n160 = xnode "Set Dynamic Data Attributes"("Signals In"=w1049, "Signal Name"="Abs P Volts") -> ("Signals Out"=w1048:dynamicdata)  [unwired: 2 in, 1 out]
    n161 = xnode "Set Dynamic Data Attributes"("Signals In"=w1052, "Signal Name"="Adjusted Abs P[Pa]") -> ("Signals Out"=w1051:dynamicdata)  [unwired: 2 in, 1 out]
    n162 = xnode "Set Dynamic Data Attributes"("Signals In"=w1058, "Signal Name"="m_dot[g/s]") -> ("Signals Out"=w1057:dynamicdata)  [unwired: 2 in, 1 out]
    n163 = xnode "Set Dynamic Data Attributes"("Signals In"=w1046, "Signal Name"="PG Temp[C]") -> ("Signals Out"=w1045:dynamicdata)  [unwired: 2 in, 1 out]
    n164 = Merge Signals(w1048, w1051, w1063, w1026, w1064, w1057, w1045, w1023, w1060, w1033, w1032) -> (w1043:dynamicdata)
    n165 = case shown="True" "Save dP data" {
      tunnel: w1043 -> [_ w1488]
      frame False {
      }
      frame True {
        n166 = call "Write To Measurement File2"("Signals"=w1488) -> ("Saving Data"=w1486:bool)  [unwired: 16 in, 2 out]
        n167 = Not(x=w1486) -> (.not. x?=w1487:bool)
        n168 = local write "Save dP data"(w1487) -> ()
      }
    }
  }
  n169 = property class="TabCtl (strict)"("BG Color"=u32 9868950 ("Color"), "FG Color"=u32 13816530 ("Color")) -> ()  [unwired: 2 in, 2 out]
  n170 = call <vilib>:"DAQmx Start Task.vi"("task/channels in"=w19) -> ("task out"=w18:refnum<k21>, "error out"=w17:errorcluster)  [unwired: 13 in]
  n171 = call <vilib>:"DAQmx Start Task.vi"("task/channels in"=w11) -> ("task out"=w10:refnum<k21>, "error out"=w9:errorcluster)  [unwired: 13 in]
  n172 = call <vilib>:"Simple Error Handler.vi"("type of dialog (OK msg:1)"=w1, "error in (no error)"=w2) -> ()  [unwired: 3 in, 5 out]
  n173 = while {
    shift-right: [w2802] -> _
    shift-left: 0.0 ("Elapsed Time (s)") -> [w2801]
    tunnel: w18 -> [w2686]
    tunnel: w17 -> [w2685]
    tunnel: [w2684] -> w16
    tunnel: [w2683] -> w15
    tunnel: w10 -> [w2663]
    tunnel: w9 -> [w2662]
    tunnel: [w2661] -> w6
    tunnel: [w2660] -> w5
    shift-right: [w2666] -> _
    shift-left: T4 {[FALSE], [FALSE], [], [], [], [], [], [], [], [], [], [], [], []} -> [w2681]
    stop <- "stop 2" stop-if-true
    w2664 = i64 100 ("Length 2")
    w2727 = T5 {"controller type"=1, "relay cycles"=3, "relay amplitude"=1.0, "control specification"=2, "PV noise level"=0.1} ("autotuning parameters")
    # "Replace with Measured Temp"
    # "Replace with Measured Temp"
    n174 = call-poly <vilib>:"DAQmx Read.vi"("task/channels in"=w2686, "error in"=w2685) -> ("task out"=w2684:refnum<k21>, "data"=w2682:dbl[], "error out"=w2683:errorcluster)  [unwired: 11 in]
    n175 = Index Array(array=w2682, index #1=1 ("index"), index #2=2 ("index"), index #3=3 ("index"), index #4=4 ("index"), index #5=5 ("index"), index #6=6 ("index"), index #7=7 ("index"), index #8=8 ("index"), index #9=9 ("index"), index #10=10 ("index"), index #11=11 ("index"), index #12=12 ("index"), index #13=13 ("index"), index #14=14 ("index")) -> (element #1=w2700:dbl, element #2=w2699:dbl, element #3=w2698:dbl, element #4=w2697:dbl, element #5=w2696:dbl, element #6=w2695:dbl, element #7=w2694:dbl, element #8=w2693:dbl, element #9=w2692:dbl, element #10=w2691:dbl, element #11=w2690:dbl, element #12=w2689:dbl, element #13=w2688:dbl, element #14=w2687:dbl)
    "T1 Measured [C]" <- w2700
    "T2 Measured [C]" <- w2699
    "T3 Measured [C]" <- w2698
    "T4 Measured [C]" <- w2697
    "T5 Measured [C]" <- w2696
    "T6 Measured [C]" <- w2695
    "T7 Measured [C]" <- w2694
    "T8 Measured [C]" <- w2693
    "T9 Measured [C]" <- w2692
    "T10 Measured [C]" <- w2691
    "T11 Measured [C]" <- w2690
    "T12 Measured [C]" <- w2689
    "T13 Measured [C]" <- w2688
    "T14 Measured [C]" <- w2687
    n176 = Build Array("T1 Setpoint [C]", w2700) -> (w2799:dbl[])
    n177 = Build Array("T2 Setpoint [C]", w2699) -> (w2793:dbl[])
    n178 = Build Array("T3 Setpoint [C]", w2698) -> (w2787:dbl[])
    n179 = Build Array("T4 Setpoint [C]", w2697) -> (w2782:dbl[])
    n180 = Build Array("T5 Setpoint [C]", w2696) -> (w2777:dbl[])
    n181 = Build Array("T6 Setpoint [C]", w2695) -> (w2772:dbl[])
    n182 = Build Array("T7 Setpoint [C]", w2694) -> (w2767:dbl[])
    n183 = Build Array("T8 Setpoint [C]", w2693) -> (w2762:dbl[])
    n184 = Build Array("T9 Setpoint [C]", w2692) -> (w2757:dbl[])
    n185 = Build Array("T10 Setpoint [C]", w2691) -> (w2752:dbl[])
    n186 = Build Array("T11 Setpoint [C]", w2690) -> (w2747:dbl[])
    n187 = Build Array("T12 Setpoint [C]", w2689) -> (w2742:dbl[])
    n188 = Build Array("T13 Setpoint [C]", w2688) -> (w2737:dbl[])
    n189 = Build Array("T14 Setpoint [C]", w2687) -> (w2732:dbl[])
    n190 = case shown="True" "PID on 8" {
      tunnel: "T8 Setpoint [C]" -> [_ w2915]
      tunnel: [0.0 ("output") w2912] -> w2759
      tunnel: w2693 -> [_ w2914]
      tunnel: "output duty cycle range 1" -> [_ w2911]
      tunnel: w2727 -> [_ w2910]
      frame False {
      }
      frame True {
        n191 = call <vilib>:"PID Autotuning.vi"("autotuning parameters"=w2910, "reinitialize? (F)"="reinitialize? (F) 10", "output range"=w2911, "PID gains"="PID gains 10", "process variable"=w2914, "setpoint"=w2915) -> ("output"=w2912:dbl)  [unwired: 2 in, 3 out]
      }
    }
    "DutyCycleCalc8" <- w2759
    n192 = case shown="True" "PID on 5" {
      tunnel: "T5 Setpoint [C]" -> [_ w2939]
      tunnel: [0.0 ("output") w2936] -> w2774
      tunnel: w2696 -> [_ w2938]
      tunnel: "output duty cycle range 1" -> [_ w2935]
      tunnel: w2727 -> [_ w2934]
      frame False {
      }
      frame True {
        n193 = call <vilib>:"PID Autotuning.vi"("autotuning parameters"=w2934, "reinitialize? (F)"="reinitialize? (F) 7", "output range"=w2935, "PID gains"="PID gains 7", "process variable"=w2938, "setpoint"=w2939) -> ("output"=w2936:dbl)  [unwired: 2 in, 3 out]
      }
    }
    "DutyCycleCalc5" <- w2774
    n194 = case shown="True" "PID on 6" {
      tunnel: "T6 Setpoint [C]" -> [_ w2931]
      tunnel: [0.0 ("output") w2928] -> w2769
      tunnel: w2695 -> [_ w2930]
      tunnel: "output duty cycle range 1" -> [_ w2927]
      tunnel: w2727 -> [_ w2926]
      frame False {
      }
      frame True {
        n195 = call <vilib>:"PID Autotuning.vi"("autotuning parameters"=w2926, "reinitialize? (F)"="reinitialize? (F) 8", "output range"=w2927, "PID gains"="PID gains 8", "process variable"=w2930, "setpoint"=w2931) -> ("output"=w2928:dbl)  [unwired: 2 in, 3 out]
      }
    }
    "DutyCycleCalc6" <- w2769
    n196 = case shown="True" "PID on" {
      tunnel: "T1 Setpoint [C]" -> [_ w2971]
      tunnel: [0.0 ("output") w2968] -> w2795
      tunnel: w2700 -> [_ w2970]
      tunnel: "output duty cycle range 1" -> [_ w2967]
      tunnel: w2727 -> [_ w2966]
      frame False {
      }
      frame True {
        n197 = call <vilib>:"PID Autotuning.vi"("autotuning parameters"=w2966, "reinitialize? (F)"="reinitialize? (F) 3", "output range"=w2967, "PID gains"="PID gains 3", "process variable"=w2970, "setpoint"=w2971) -> ("output"=w2968:dbl)  [unwired: 2 in, 3 out]
      }
    }
    "DutyCycleCalc1" <- w2795
    n198 = case shown="True" "PID on 7" {
      tunnel: "T7 Setpoint [C]" -> [_ w2923]
      tunnel: [0.0 ("output") w2920] -> w2764
      tunnel: w2694 -> [_ w2922]
      tunnel: "output duty cycle range 1" -> [_ w2919]
      tunnel: w2727 -> [_ w2918]
      frame False {
      }
      frame True {
        n199 = call <vilib>:"PID Autotuning.vi"("autotuning parameters"=w2918, "reinitialize? (F)"="reinitialize? (F) 9", "output range"=w2919, "PID gains"="PID gains 9", "process variable"=w2922, "setpoint"=w2923) -> ("output"=w2920:dbl)  [unwired: 2 in, 3 out]
      }
    }
    "DutyCycleCalc7" <- w2764
    n200 = case shown="True" "PID on 3" {
      tunnel: "T3 Setpoint [C]" -> [_ w2955]
      tunnel: [0.0 ("output") w2952] -> w2784
      tunnel: w2698 -> [_ w2954]
      tunnel: "output duty cycle range 1" -> [_ w2951]
      tunnel: w2727 -> [_ w2950]
      frame False {
      }
      frame True {
        n201 = call <vilib>:"PID Autotuning.vi"("autotuning parameters"=w2950, "reinitialize? (F)"="reinitialize? (F) 5", "output range"=w2951, "PID gains"="PID gains 5", "process variable"=w2954, "setpoint"=w2955) -> ("output"=w2952:dbl)  [unwired: 2 in, 3 out]
      }
    }
    "DutyCycleCalc3" <- w2784
    n202 = case shown="True" "PID on 4" {
      tunnel: "T4 Setpoint [C]" -> [_ w2947]
      tunnel: [0.0 ("output") w2944] -> w2779
      tunnel: w2697 -> [_ w2946]
      tunnel: "output duty cycle range 1" -> [_ w2943]
      tunnel: w2727 -> [_ w2942]
      frame False {
      }
      frame True {
        n203 = call <vilib>:"PID Autotuning.vi"("autotuning parameters"=w2942, "reinitialize? (F)"="reinitialize? (F) 6", "output range"=w2943, "PID gains"="PID gains 6", "process variable"=w2946, "setpoint"=w2947) -> ("output"=w2944:dbl)  [unwired: 2 in, 3 out]
      }
    }
    "DutyCycleCalc4" <- w2779
    n204 = case shown="True" "PID on 9" {
      tunnel: "T9 Setpoint [C]" -> [_ w2907]
      tunnel: [0.0 ("output") w2904] -> w2754
      tunnel: w2692 -> [_ w2906]
      tunnel: "output duty cycle range 1" -> [_ w2903]
      tunnel: w2727 -> [_ w2902]
      frame False {
      }
      frame True {
        n205 = call <vilib>:"PID Autotuning.vi"("autotuning parameters"=w2902, "reinitialize? (F)"="reinitialize? (F) 11", "output range"=w2903, "PID gains"="PID gains 11", "process variable"=w2906, "setpoint"=w2907) -> ("output"=w2904:dbl)  [unwired: 2 in, 3 out]
      }
    }
    "DutyCycleCalc9" <- w2754
    n206 = case shown="True" "PID on 2" {
      tunnel: "T2 Setpoint [C]" -> [_ w2963]
      tunnel: [0.0 ("output") w2960] -> w2790
      tunnel: w2699 -> [_ w2962]
      tunnel: "output duty cycle range 1" -> [_ w2959]
      tunnel: w2727 -> [_ w2958]
      frame False {
      }
      frame True {
        n207 = call <vilib>:"PID Autotuning.vi"("autotuning parameters"=w2958, "reinitialize? (F)"="reinitialize? (F) 4", "output range"=w2959, "PID gains"="PID gains 4", "process variable"=w2962, "setpoint"=w2963) -> ("output"=w2960:dbl)  [unwired: 2 in, 3 out]
      }
    }
    "DutyCycleCalc2" <- w2790
    n208 = case shown="True" "PID on 10" {
      tunnel: "T10 Setpoint [C]" -> [_ w2899]
      tunnel: [0.0 ("output") w2896] -> w2749
      tunnel: w2691 -> [_ w2898]
      tunnel: "output duty cycle range 1" -> [_ w2895]
      tunnel: w2727 -> [_ w2894]
      frame False {
      }
      frame True {
        n209 = call <vilib>:"PID Autotuning.vi"("autotuning parameters"=w2894, "reinitialize? (F)"="reinitialize? (F) 12", "output range"=w2895, "PID gains"="PID gains 12", "process variable"=w2898, "setpoint"=w2899) -> ("output"=w2896:dbl)  [unwired: 2 in, 3 out]
      }
    }
    "DutyCycleCalc10" <- w2749
    n210 = case shown="True" "PID on 14" {
      tunnel: "T14 Setpoint [C]" -> [_ w2867]
      tunnel: [0.0 ("output") w2864] -> w2729
      tunnel: w2687 -> [_ w2866]
      tunnel: "output duty cycle range 1" -> [_ w2863]
      tunnel: w2727 -> [_ w2862]
      frame False {
      }
      frame True {
        n211 = call <vilib>:"PID Autotuning.vi"("autotuning parameters"=w2862, "reinitialize? (F)"="reinitialize? (F) 16", "output range"=w2863, "PID gains"="PID gains 16", "process variable"=w2866, "setpoint"=w2867) -> ("output"=w2864:dbl)  [unwired: 2 in, 3 out]
      }
    }
    "DutyCycleCalc14" <- w2729
    n212 = case shown="True" "PID on 12" {
      tunnel: "T12 Setpoint [C]" -> [_ w2883]
      tunnel: [0.0 ("output") w2880] -> w2739
      tunnel: w2689 -> [_ w2882]
      tunnel: "output duty cycle range 1" -> [_ w2879]
      tunnel: w2727 -> [_ w2878]
      frame False {
      }
      frame True {
        n213 = call <vilib>:"PID Autotuning.vi"("autotuning parameters"=w2878, "reinitialize? (F)"="reinitialize? (F) 14", "output range"=w2879, "PID gains"="PID gains 14", "process variable"=w2882, "setpoint"=w2883) -> ("output"=w2880:dbl)  [unwired: 2 in, 3 out]
      }
    }
    "DutyCycleCalc12" <- w2739
    n214 = case shown="True" "PID on 11" {
      tunnel: "T11 Setpoint [C]" -> [_ w2891]
      tunnel: [0.0 ("output") w2888] -> w2744
      tunnel: w2690 -> [_ w2890]
      tunnel: "output duty cycle range 1" -> [_ w2887]
      tunnel: w2727 -> [_ w2886]
      frame False {
      }
      frame True {
        n215 = call <vilib>:"PID Autotuning.vi"("autotuning parameters"=w2886, "reinitialize? (F)"="reinitialize? (F) 13", "output range"=w2887, "PID gains"="PID gains 13", "process variable"=w2890, "setpoint"=w2891) -> ("output"=w2888:dbl)  [unwired: 2 in, 3 out]
      }
    }
    "DutyCycleCalc11" <- w2744
    n216 = case shown="True" "PID on 13" {
      tunnel: "T13 Setpoint [C]" -> [_ w2875]
      tunnel: [0.0 ("output") w2872] -> w2734
      tunnel: w2688 -> [_ w2874]
      tunnel: "output duty cycle range 1" -> [_ w2871]
      tunnel: w2727 -> [_ w2870]
      frame False {
      }
      frame True {
        n217 = call <vilib>:"PID Autotuning.vi"("autotuning parameters"=w2870, "reinitialize? (F)"="reinitialize? (F) 15", "output range"=w2871, "PID gains"="PID gains 15", "process variable"=w2874, "setpoint"=w2875) -> ("output"=w2872:dbl)  [unwired: 2 in, 3 out]
      }
    }
    "DutyCycleCalc13" <- w2734
    n218 = Array To Cluster(array=w2793) -> (cluster=→"T2":cluster{"[0]":dbl, "[1]":dbl})
    n219 = Array To Cluster(array=w2787) -> (cluster=→"T3":cluster{"[0]":dbl, "[1]":dbl})
    n220 = Array To Cluster(array=w2782) -> (cluster=→"T4":cluster{"[0]":dbl, "[1]":dbl})
    n221 = Array To Cluster(array=w2777) -> (cluster=→"T5":cluster{"[0]":dbl, "[1]":dbl})
    n222 = Array To Cluster(array=w2772) -> (cluster=→"T6":cluster{"[0]":dbl, "[1]":dbl})
    n223 = Array To Cluster(array=w2767) -> (cluster=→"T7":cluster{"[0]":dbl, "[1]":dbl})
    n224 = Array To Cluster(array=w2762) -> (cluster=→"T8":cluster{"[0]":dbl, "[1]":dbl})
    n225 = Array To Cluster(array=w2757) -> (cluster=→"T9":cluster{"[0]":dbl, "[1]":dbl})
    n226 = Array To Cluster(array=w2752) -> (cluster=→"T10":cluster{"[0]":dbl, "[1]":dbl})
    n227 = Array To Cluster(array=w2747) -> (cluster=→"T11":cluster{"[0]":dbl, "[1]":dbl})
    n228 = Array To Cluster(array=w2742) -> (cluster=→"T12":cluster{"[0]":dbl, "[1]":dbl})
    n229 = Array To Cluster(array=w2737) -> (cluster=→"T13":cluster{"[0]":dbl, "[1]":dbl})
    n230 = Array To Cluster(array=w2732) -> (cluster=→"T14":cluster{"[0]":dbl, "[1]":dbl})
    n231 = Array To Cluster(array=w2799) -> (cluster=→"T1":cluster{"[0]":dbl, "[1]":dbl})
    n232 = To Quad Integer(1:w2790) -> (0:w2789:i64)
    n233 = To Quad Integer(1:w2759) -> (0:w2721:i64)
    n234 = To Quad Integer(1:w2774) -> (0:w2724:i64)
    n235 = To Quad Integer(1:w2769) -> (0:w2723:i64)
    n236 = To Quad Integer(1:w2795) -> (0:w2796:i64)
    n237 = To Quad Integer(1:w2764) -> (0:w2722:i64)
    n238 = To Quad Integer(1:w2784) -> (0:w2726:i64)
    n239 = To Quad Integer(1:w2779) -> (0:w2725:i64)
    n240 = To Quad Integer(1:w2754) -> (0:w2720:i64)
    n241 = To Quad Integer(1:w2749) -> (0:w2719:i64)
    n242 = To Quad Integer(1:w2729) -> (0:w2715:i64)
    n243 = To Quad Integer(1:w2744) -> (0:w2718:i64)
    n244 = To Quad Integer(1:w2734) -> (0:w2716:i64)
    n245 = To Quad Integer(1:w2739) -> (0:w2717:i64)
    n246 = Unbundle(w2681) -> (w2659:bool[], w2665:bool[])  [unwired: 12 out]
    n247 = for {
      N: w2664 -> [_]
      tunnel: w2796 -> [w2860]
      tunnel: [w2859] -> w2680 mode=indexing
      tunnel: w2789 -> [w2858]
      tunnel: [w2857] -> w2679 mode=indexing
      tunnel: w2726 -> [w2856]
      tunnel: w2725 -> [w2854]
      tunnel: w2724 -> [w2853]
      tunnel: w2723 -> [w2852]
      tunnel: w2722 -> [w2851]
      tunnel: w2721 -> [w2850]
      tunnel: w2720 -> [w2849]
      tunnel: w2719 -> [w2848]
      tunnel: w2718 -> [w2847]
      tunnel: w2717 -> [w2846]
      tunnel: w2716 -> [w2845]
      tunnel: w2715 -> [w2844]
      tunnel: [w2843] -> w2678 mode=indexing
      tunnel: [w2842] -> w2677 mode=indexing
      tunnel: [w2841] -> w2676 mode=indexing
      tunnel: [w2840] -> w2675 mode=indexing
      tunnel: [w2839] -> w2674 mode=indexing
      tunnel: [w2838] -> w2673 mode=indexing
      tunnel: [w2837] -> w2672 mode=indexing
      tunnel: [w2836] -> w2671 mode=indexing
      tunnel: [w2835] -> w2670 mode=indexing
      tunnel: [w2834] -> w2669 mode=indexing
      tunnel: [w2833] -> w2668 mode=indexing
      tunnel: [w2832] -> w2667 mode=indexing
      i -> [w2855]
      n248 = Greater?(x=w2858, y=w2855) -> (0:w2857:bool)
      n249 = Greater?(x=w2850, y=w2855) -> (0:w2838:bool)
      n250 = Greater?(x=w2853, y=w2855) -> (0:w2841:bool)
      n251 = Greater?(x=w2852, y=w2855) -> (0:w2840:bool)
      n252 = Greater?(x=w2860, y=w2855) -> (0:w2859:bool)
      n253 = Greater?(x=w2851, y=w2855) -> (0:w2839:bool)
      n254 = Greater?(x=w2856, y=w2855) -> (0:w2843:bool)
      n255 = Greater?(x=w2854, y=w2855) -> (0:w2842:bool)
      n256 = Greater?(x=w2849, y=w2855) -> (0:w2837:bool)
      n257 = Greater?(x=w2848, y=w2855) -> (0:w2836:bool)
      n258 = Greater?(x=w2844, y=w2855) -> (0:w2832:bool)
      n259 = Greater?(x=w2847, y=w2855) -> (0:w2835:bool)
      n260 = Greater?(x=w2845, y=w2855) -> (0:w2833:bool)
      n261 = Greater?(x=w2846, y=w2855) -> (0:w2834:bool)
    }
    n262 = for {
      N: w2664 -> [_]
      tunnel: w2665 -> [w2824] mode=indexing
      tunnel: [w2827] -> w2661
      tunnel: [w2826] -> w2660
      tunnel: w2663 -> [w2830]
      tunnel: w2662 -> [w2829]
      tunnel: w2659 -> [w2825] mode=indexing
      n263 = Build Array(w2825, w2824) -> (w2828:bool[])
      n264 = Wait (ms)(milliseconds to wait=u32 10) -> ()  [unwired: 1 out]
      n265 = call-poly <vilib>:"DAQmx Write.vi"("task/channels in"=w2830, "data"=w2828, "error in"=w2829) -> ("task out"=w2827:refnum<k21>, "error out"=w2826:errorcluster)  [unwired: 10 in, 1 out]
      "WinOn 2" <- w2824
      "WinOn 1" <- w2825
    }
    n266 = disable-structure shown="Disabled" {
      disable-tunnel: w2664 -> [w2818 _]
      disable-tunnel: w2680 -> [w2817 _]
      disable-tunnel: w2679 -> [w2816 _]
      disable-tunnel: w2678 -> [w2815 _]
      disable-tunnel: w2677 -> [w2814 _]
      disable-tunnel: w2676 -> [w2813 _]
      disable-tunnel: w2675 -> [w2812 _]
      disable-tunnel: w2674 -> [w2811 _]
      disable-tunnel: w2673 -> [w2810 _]
      disable-tunnel: w2672 -> [w2809 _]
      disable-tunnel: w2671 -> [w2808 _]
      disable-tunnel: w2670 -> [w2807 _]
      disable-tunnel: w2669 -> [w2806 _]
      disable-tunnel: w2668 -> [w2805 _]
      disable-tunnel: w2667 -> [w2804 _]
      frame Disabled {
        n267 = for {
          N: w2818 -> [_]
          tunnel: w2817 -> [_] mode=indexing
          tunnel: w2816 -> [w2819] mode=indexing
          tunnel: w2815 -> [_] mode=indexing
          tunnel: w2814 -> [_] mode=indexing
          tunnel: w2813 -> [_] mode=indexing
          tunnel: w2812 -> [_] mode=indexing
          tunnel: w2811 -> [_] mode=indexing
          tunnel: w2810 -> [_] mode=indexing
          tunnel: w2809 -> [_] mode=indexing
          tunnel: w2808 -> [_] mode=indexing
          tunnel: w2807 -> [_] mode=indexing
          tunnel: w2806 -> [_] mode=indexing
          tunnel: w2805 -> [_] mode=indexing
          tunnel: w2804 -> [_] mode=indexing
          tunnel: [w2821] -> _
          tunnel: [w2820] -> _
          n268 = Build Array(w2819) -> (w2822:bool[])
          n269 = Wait (ms)(milliseconds to wait=u32 10) -> ()  [unwired: 1 out]
          n270 = call-poly <vilib>:"DAQmx Write.vi"("data"=w2822) -> ("task out"=w2821:refnum<k21>, "error out"=w2820:errorcluster)  [unwired: 12 in, 1 out]
        }
      }
      frame Enabled {
      }
    }
    n271 = Bundle(w2680, w2679, w2678, w2677, w2676, w2675, w2674, w2673, w2672, w2671, w2670, w2669, w2668, w2667) -> (w2666:T4)  [unwired: 1 in]
    n272 = call "Elapsed Time"() -> ("Elapsed Time (s)"=w2802:dbl)  [unwired: 12 in, 7 out]
    n273 = Wait (ms)(milliseconds to wait=u32 1000) -> ()  [unwired: 1 out]
    n274 = Subtract(x=w2802, y=w2801) -> (x-y=→"Waveform Chart" →"Elapsed Time (s)":dbl)
  }
  n275 = call <vilib>:"DAQmx Stop Task.vi"("task/channels in"=w16, "error in"=w15) -> ("task out"=w22:refnum<k21>, "error out"=w21:errorcluster)  [unwired: 12 in]
  n276 = call <vilib>:"DAQmx Clear Task.vi"("task in"=w22, "error in"=w21) -> ("error out"=→"error out":errorcluster)  [unwired: 13 in]
  n277 = call-poly <vilib>:"DAQmx Write.vi"("task/channels in"=w6, "data"=bool[] [FALSE], "error in"=w5) -> ("task out"=w8:refnum<k21>, "error out"=w7:errorcluster)  [unwired: 10 in, 1 out]
  n278 = call <vilib>:"DAQmx Stop Task.vi"("task/channels in"=w8, "error in"=w7) -> ("task out"=w14:refnum<k21>, "error out"=w13:errorcluster)  [unwired: 12 in]
  n279 = call <vilib>:"DAQmx Clear Task.vi"("task in"=w14, "error in"=w13) -> ("error out"=→"error out 2":errorcluster)  [unwired: 13 in]
